vi "Derivative (DBL).vi"(2 "initialize":bool, 3 "dt":dbl=1e-09 min=1e-09 format="%.6f", 4 "initial condition":dbl format="%.2f", 5 "input point":dbl format="%.2f") -> (1 "output point":dbl format="%.2f")   [LabVIEW 2020, in "NI_AdvCtrl_continuous linear.lvlib"]
doc: "LabVIEW no longer supports this VI. You can obtain similar functionality by installing the LabVIEW Simulation Module.\n\nCalculates the derivative of a continuous signal, where the formula output(n)=(input(n)-input(n-1))/dt is used. This element is a specific transfer function with H(s)=s."
uses:
  <vilib>/addons/control/advanced/NI_AdvCtrl_continuous linear.lvlib
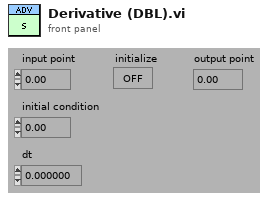
[diagram p1: front panel]
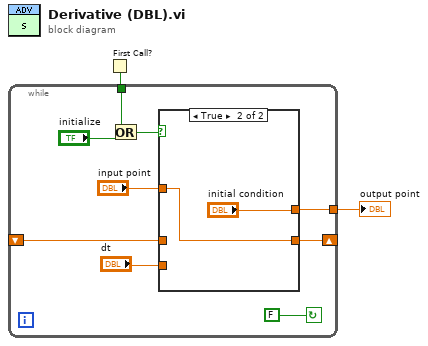
[diagram p0: block diagram]
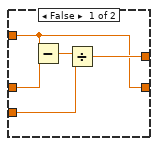
[diagram p2: hidden frame]
diagram:
  n1 = First Call?() -> (First Call?: T/F=w1:bool)
  n2 = while {
    tunnel: w1 -> [w5]
    tunnel: [w8] -> w2
    shift-left: _ -> [w10]
    shift-right: [w11] -> _
    stop <- FALSE continue-if-true
    n3 = Or(x=w5, y="initialize") -> (x .or. y?=w4:bool)
    n4 = case shown="True" w4 {
      tunnel: [w13 w18] -> w11
      tunnel: w10 -> [w16 _]
      tunnel: "input point" -> [w13 w18]
      tunnel: [w14 "initial condition"] -> w8
      tunnel: "dt" -> [w12 _]
      frame False {
        n5 = Subtract(x=w13, y=w16) -> (x-y=w15:dbl)
        n6 = Divide(x=w15, y=w12) -> (x/y=w14:dbl)
      }
      frame True {
      }
    }
  }
  "output point" <- w2
